vi "Drive Code.vi"() -> ()   [LabVIEW 2013]
uses:
  <vilib>/Rock Robotics/WPI/Joystick/WPI_JoystickGetSetRefNum.vi
  Robot Global Data.vi
  Globals/Data for Dashboard.vi
panel:
  out "Flip Axes?":bool
  out "Angular Rate":dbl
  out "Angle":dbl=230.22186489896953
  in  "Gyro input":dbl=-0.05 format="%#_13g"
  out "Gyro":dbl=-0.0
  in  "Gyro turn":dbl=1.0
  out "Left Motor":dbl=-4.843459373818121e-07
  out "Right Motor":dbl=-4.920339681339045e-07
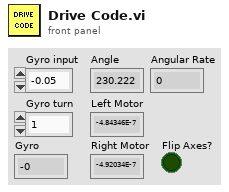
[diagram p1: front panel]
types:
  T1 = typedef "WPI_MotorControlDeviceRef.ctl" = cluster{"DeviceStatus":errorcluster, "Type":enum16{"PWM", "CAN"}, "PWM":cluster{"Digital Module":T2, "PWM Channel":T3, "DeadBand":T4}, "CAN":cluster{"Device Number":u8, "Control Mode":T5, "Semaphore":T6, "Max Vout":dbl}, "Invert":bool, "TransformRef":T7, "InvTransformRef":T7}
  T2 = typedef "FPGA_TypedefDigitalModule.ctl" = enum16{"Digital Module 1", "Digital Module 2"}
  T3 = typedef "FPGA_DIOPWMChannel.ctl" = enum8{"PWM 1", "PWM 2", "PWM 3", "PWM 4", "PWM 5", "PWM 6", "PWM 7", "PWM 8", "PWM 9", "PWM 10", "Invalid"}
  T4 = typedef "WPI_PWMDeadband.ctl" = cluster{"Name":string, "maxPositivePwm":i32, "minPositivePwm":i32, "centerPwm":i32, "maxNegativePwm":i32, "minNegativePwm":i32, "angularRange":u16}
  T5 = typedef "WPI_CANJaguar_ControlMode.ctl" = enum8{"Percent VBus", "Current", "Speed", "Position", "Voltage"}
  T6 = typedef "Semaphore RefNum" = refnum<k1>
  T7 = typedef "WPI_PWMTransform_ConPane.ctl" = refnum<vi>
  T8 = typedef "WPI_JoystickDevRef.ctl" = cluster{"Device":T9}
  T9 = typedef "WPI_JoystickDeviceEnum.ctl" = enum16{"USB 1", "USB 2", "USB 3", "USB 4", "Kinect 1", "Kinect 2"}
  T10 = typedef "WPI_I2CDevRef.ctl" = cluster{"DevStatus":errorcluster, "Digital Module":T2, "Device Address":u8}
  T11 = typedef "WPI_DigitalOutputDevRef.ctl" = cluster{"Digital Module":T2, "DIO Channel":T12, "DevStatus":errorcluster}
  T12 = typedef "FPGA_DIOChannel.ctl" = enum8{"DIO 1", "DIO 2", "DIO 3", "DIO 4", "DIO 5", "DIO 6", "DIO 7", "DIO 8", "DIO 9", "DIO 10", "DIO 11", "DIO 12", "DIO 13", "DIO 14", "Invalid"}
  T13 = typedef "WPI_JoystickButtonState.ctl" = cluster{"Button 1":bool, "Button 2":bool, "Button 3":bool, "Button 4":bool, "Button 5":bool, "Button 6":bool, "Button 7":bool, "Button 8":bool, "Button 9":bool, "Button 10":bool, "Button 11":bool, "Button 12":bool}
  T14 = typedef "WPI_DriverStationRobotMode2.ctl" = enum16{"Autonomous Disabled", "Autonomous Enabled", "Teleop Disabled", "Teleop Enabled", "Timeout", "Finish", "Test Disabled", "Test Enabled"}
  T15 = cluster{"axis 1 (x)":dbl, "axis 2 (y)":dbl, "axis 3 (throttle)":dbl, "axis 4":dbl, "axis 5":dbl, "axis 6":dbl}
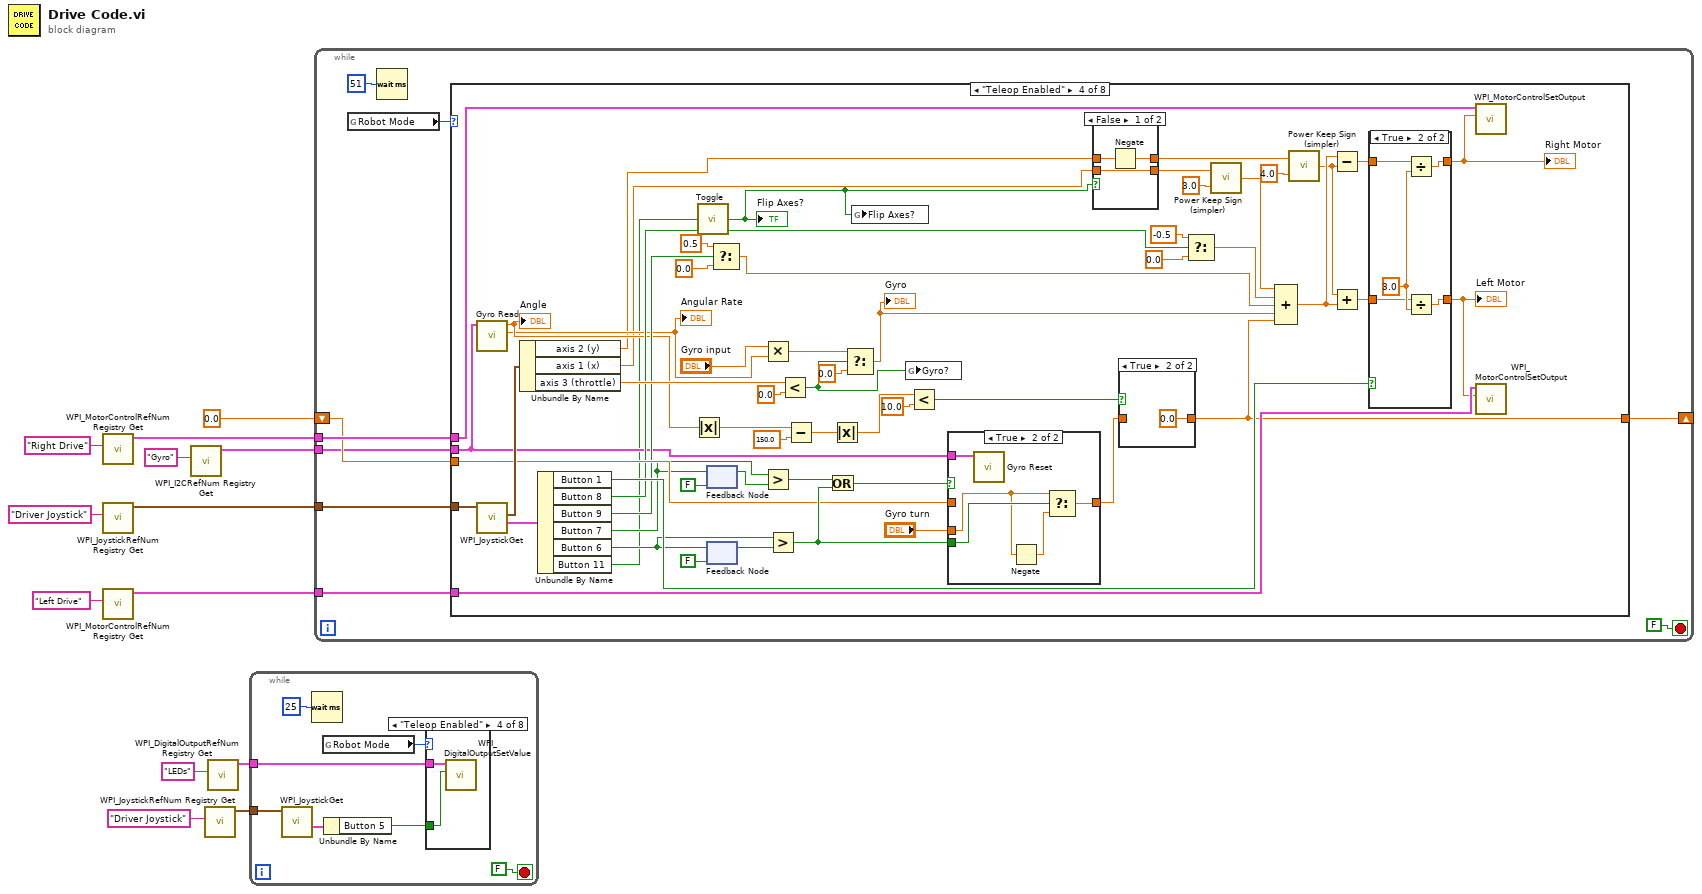
[diagram p0: block diagram]
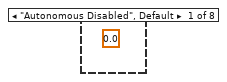
[diagram p9: hidden frame]
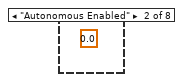
[diagram p10: hidden frame]
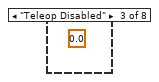
[diagram p11: hidden frame]
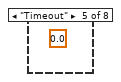
[diagram p16: hidden frame]
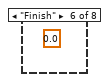
[diagram p17: hidden frame]
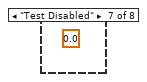
[diagram p18: hidden frame]
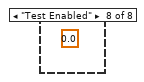
[diagram p19: hidden frame]
diagram:
  n1 = call <vilib>:"WPI_MotorControlRefNum Registry Get.vi"("refnum name"="Right Drive") -> ("MotorControlDevRef"=w10:T1)  [unwired: 9 in, 1 out]
  n2 = call <vilib>:"WPI_JoystickRefNum Registry Get.vi"("refnum name"="Driver Joystick") -> ("JoystickDevRef"=w13:T8)  [unwired: 9 in, 1 out]
  n3 = call <vilib>:"WPI_MotorControlRefNum Registry Get.vi"("refnum name"="Left Drive") -> ("MotorControlDevRef"=w7:T1)  [unwired: 9 in, 1 out]
  n4 = call <vilib>:"WPI_I2CRefNum Registry Get.vi"("refnum name"="Gyro") -> ("I2CDevRef"=w5:T10)  [unwired: 9 in, 1 out]
  n5 = call <vilib>:"WPI_JoystickRefNum Registry Get.vi"("refnum name"="Driver Joystick") -> ("JoystickDevRef"=w3:T8)  [unwired: 9 in, 1 out]
  n6 = call <vilib>:"WPI_DigitalOutputRefNum Registry Get.vi"("refnum name"="LEDs") -> ("DigitalOutputDevRef"=w2:T11)  [unwired: 9 in, 1 out]
  n7 = while {
    tunnel: w3 -> [w18]
    tunnel: w2 -> [w15]
    stop <- FALSE stop-if-true
    n8 = call <vilib>:"WPI_JoystickGet.vi"("JoystickDevRef"=w18) -> ("Buttons"=w17:T13)  [unwired: 4 in, 2 out]
    n9 = Wait (ms)(milliseconds to wait=u32 25) -> ()  [unwired: 1 out]
    n10 = global read "Robot Global Data.vi" "Robot Mode"() -> (w14:T14)
    n11 = Unbundle By Name(w17) -> ("Button 5"=w16:bool)
    n12 = case shown="\"Teleop Enabled\"" w14 {
      tunnel: w16 -> [_ _ _ w22 _ _ _ _]
      tunnel: w15 -> [_ _ _ w21 _ _ _ _]
      frame "Autonomous Disabled", Default {
      }
      frame "Autonomous Enabled" {
      }
      frame "Teleop Disabled" {
      }
      frame "Teleop Enabled" {
        n13 = call <vilib>:"WPI_DigitalOutputSetValue.vi"("Value"=w22, "DigitalOutputDevRef"=w21) -> ()  [unwired: 8 in, 2 out]
      }
      frame "Timeout" {
      }
      frame "Finish" {
      }
      frame "Test Disabled" {
      }
      frame "Test Enabled" {
      }
    }
  }
  n14 = while {
    tunnel: w13 -> [w31]
    tunnel: w10 -> [w30]
    shift-right: [w25] -> _
    shift-left: 0.0 ("f") -> [w26]
    tunnel: w7 -> [w24]
    tunnel: w5 -> [w23]
    stop <- FALSE stop-if-true
    n15 = global read "Robot Global Data.vi" "Robot Mode"() -> (w29:T14)
    n16 = Wait (ms)(milliseconds to wait=u32 51) -> ()  [unwired: 1 out]
    n17 = case shown="\"Teleop Enabled\"" w29 {
      tunnel: w31 -> [_ _ _ w89 _ _ _ _]
      tunnel: w30 -> [_ _ _ w87 _ _ _ _]
      tunnel: w26 -> [_ _ _ w57 _ _ _ _]
      tunnel: [_ _ _ w41 _ _ _ _] -> w25
      tunnel: w24 -> [_ _ _ w55 _ _ _ _]
      tunnel: w23 -> [_ _ _ w42 _ _ _ _]
      frame "Autonomous Disabled", Default {
        (unwired) 0.0 ("t")
      }
      frame "Autonomous Enabled" {
        (unwired) 0.0 ("t")
      }
      frame "Teleop Disabled" {
        (unwired) 0.0 ("t")
      }
      frame "Teleop Enabled" {
        n18 = call "Gyro Read.vi"("I2CDevRef In"=w42) -> ("Angular Rate"=w44:dbl, "Angle"=w45:dbl)  [unwired: 9 in]
        "Angle" <- w45
        "Angular Rate" <- w44
        n19 = call <vilib>:"WPI_JoystickGet.vi"("JoystickDevRef"=w89) -> ("Buttons"=w84:T13, "Axes"=w88:T15)  [unwired: 4 in, 1 out]
        n20 = Unbundle By Name(w88) -> ("axis 2 (y)"=w36:dbl, "axis 1 (x)"=w38:dbl, "axis 3 (throttle)"=w72:dbl)
        n21 = Unbundle By Name(w84) -> ("Button 1"=w81:bool, "Button 8"=w50:bool, "Button 9"=w53:bool, "Button 7"=w54:bool, "Button 6"=w52:bool, "Button 11"=w40:bool)
        n22 = Absolute Value(x=w45) -> (abs(x)=w66:dbl)
        n23 = call "Toggle.vi"("Input"=w40) -> ("Output"=w35:bool)
        "Flip Axes?" <- w35
        n24 = feedback #1(FALSE ("Boolean")) -> (w58:bool)
        n25 = feedback-in #1(w54) -> ()
        n26 = feedback #2(FALSE ("Boolean")) -> (w61:bool)
        n27 = feedback-in #2(w52) -> ()
        n28 = Select(t=0.5, s=w53, f=0.0) -> (s? t:f=w48:dbl)
        n29 = Multiply(x="Gyro input", y=w44) -> (x*y=w46:dbl)
        n30 = Greater?(x=w54, y=w58) -> (0:w62:bool)
        n31 = Greater?(x=w52, y=w61) -> (0:w65:bool)
        n32 = Less?(x=w72, y=0.0) -> (x < y?=w34:bool)
        n33 = Subtract(x=w66, y=150.0) -> (x-y=w68:dbl)
        n34 = Or(x=w62, y=w65) -> (x .or. y?=w63:bool)
        n35 = Absolute Value(x=w68) -> (abs(x)=w56:dbl)
        n36 = Select(t=w46, s=w34, f=0.0 ("t")) -> (s? t:f=w43:dbl)
        "Gyro" <- w43
        n37 = global write "Data for Dashboard.vi" "Flip Axes?"(w35) -> ()
        n38 = global write "Data for Dashboard.vi" "Gyro?"(w34) -> ()
        n39 = Less?(x=w56, y=10.0) -> (x < y?=w70:bool)
        n40 = case shown="True" w63 {
          tunnel: "Gyro turn" -> [_ w101]
          tunnel: w65 -> [_ w102]
          tunnel: [w97 w99] -> w71
          tunnel: w57 -> [w97 _]
          tunnel: w42 -> [_ w98]
          frame False {
          }
          frame True {
            n41 = call "Gyro Reset.vi"("I2CDevRef"=w98) -> ()  [unwired: 10 in, 1 out]
            n42 = Negate(x=w101) -> (-x=w100:dbl)
            n43 = Select(t=w101, s=w102, f=w100) -> (s? t:f=w99:dbl)
          }
        }
        n44 = case shown="False" w35 {
          tunnel: w36 -> [w91 w93]
          tunnel: [w90 w93] -> w39
          tunnel: w38 -> [w92 w94]
          tunnel: [w92 w94] -> w37
          frame False {
            n45 = Negate(x=w91) -> (-x=w90:dbl)
          }
          frame True {
          }
        }
        n46 = case shown="True" w70 {
          tunnel: [w95 0.0 ("Gyro turn")] -> w41
          tunnel: w71 -> [w95 _]
          frame False {
          }
          frame True {
          }
        }
        n47 = Select(t=-0.5, s=w50, f=0.0) -> (s? t:f=w49:dbl)
        n48 = call "Power Keep Sign (simpler).vi"("Power"=3.0, "In"=w37) -> ("Out"=w74:dbl)
        n49 = Compound Arithmetic op=ADD(w74, w49, w48, w43, w41) -> (w80:dbl)
        n50 = call "Power Keep Sign (simpler).vi"("Power"=4.0, "In"=w39) -> ("Out"=w79:dbl)
        n51 = Subtract(x=w80, y=w79) -> (x-y=w83:dbl)
        n52 = Add(x=w79, y=w80) -> (x+y=w82:dbl)
        n53 = case shown="True" w81 {
          tunnel: w83 -> [w104 w109]
          tunnel: [w104 w107] -> w32
          tunnel: w82 -> [w103 w105]
          tunnel: [w103 w108] -> w33
          frame False {
          }
          frame True {
            w106 = 3.0 ("y")
            n54 = Divide(x=w109, y=w106) -> (x/y=w107:dbl)
            n55 = Divide(x=w105, y=w106) -> (x/y=w108:dbl)
          }
        }
        "Left Motor" <- w33
        "Right Motor" <- w32
        n56 = call <vilib>:"WPI_MotorControlSetOutput.vi"("Output"=w32, "MotorControlDevRef"=w87) -> ()  [unwired: 7 in, 3 out]
        n57 = call <vilib>:"WPI_MotorControlSetOutput.vi"("Output"=w33, "MotorControlDevRef"=w55) -> ()  [unwired: 7 in, 3 out]
      }
      frame "Timeout" {
        (unwired) 0.0 ("t")
      }
      frame "Finish" {
        (unwired) 0.0 ("t")
      }
      frame "Test Disabled" {
        (unwired) 0.0 ("t")
      }
      frame "Test Enabled" {
        (unwired) 0.0 ("t")
      }
    }
  }
